vi "ParseObject.vi"(8 "error in (no error)":errorcluster, 10 "Tag In":string, 11 "Object_XML":string) -> (0 "error out":errorcluster, 3 "Array":T1[](array[typedef]))   [LabVIEW 2022 SP3, in "Object_Editor.lvlib" / "Object_Editor.lvclass"]
uses:
  Object_Editor.lvclass
  TreeItem.ctl
  ItemType.ctl
  <vilib>/xml/Load XML String.vi
  <vilib>/xml/Close Reference(Node).vi
  <vilib>/xml/NI_XML.lvlib
  <resource>/objmgr/DOMUserDefRef.rc
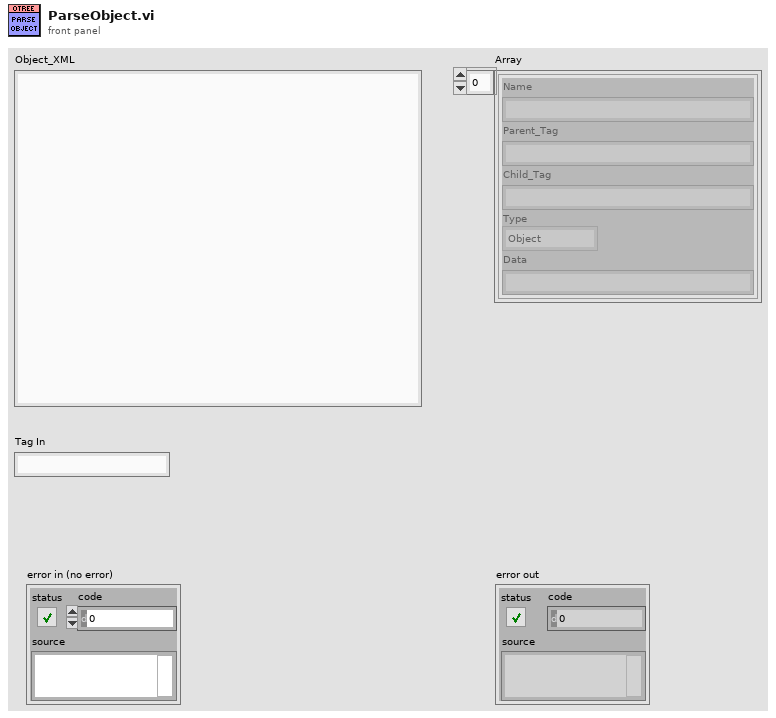
[diagram p1: front panel]
types:
  T1 = typedef "Object_Editor.lvlib/Object_Editor.lvclass/TreeItem.ctl" = cluster{"Name":string, "Parent_Tag":string, "Child_Tag":string, "Type":T2, "Data":string}
  T2 = typedef "Object_Editor.lvlib/Object_Editor.lvclass/ItemType.ctl" = enum16{"Object", "Ancestor"}
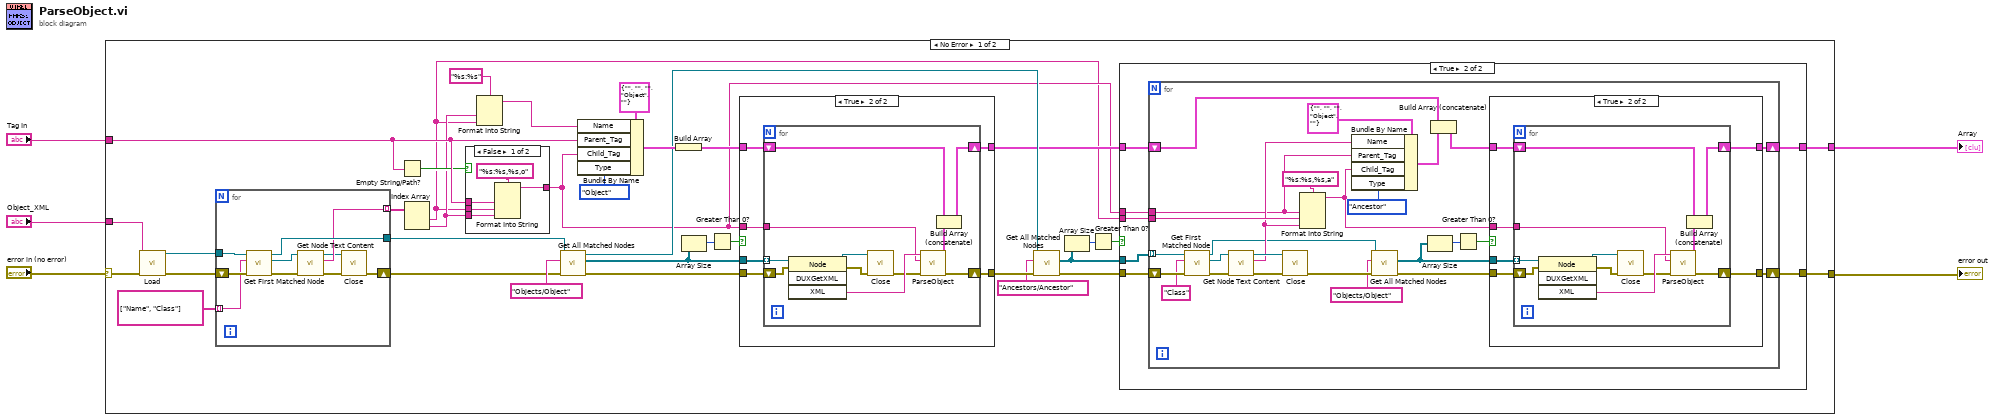
[diagram p0: block diagram]
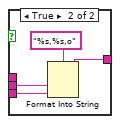
[diagram p4: hidden frame]
diagram:
  n1 = case shown="No Error" "error in (no error)" {
    selector: "error in (no error)" -> [w39 w132]
    tunnel: "Object_XML" -> [w38 _]
    tunnel: "Tag In" -> [w25 _]
    tunnel: [w12 w132] -> w1
    tunnel: [w11 _] -> w2
    frame No Error {
      n2 = call-poly <vilib>:"Load.vi"("XML string"=w38, "error in (no error)"=w39) -> ("DOM document out"=w36:refnum<k20>, "error out"=w37:errorcluster)  [unwired: 11 in, 1 out]
      n3 = for {
        tunnel: [w108] -> w30
        tunnel: [w107] -> w26 mode=indexing
        shift-right: [w104] -> w27
        shift-left: w37 -> [w112]
        tunnel: w36 -> [w111]
        tunnel: string[] ["Name", "Class"] -> [w106] mode=indexing
        n4 = call <vilib>:"Get First Matched Node.vi"("error in (no error)"=w112, "XPath expression"=w106, "node in"=w111) -> ("error out"=w110:errorcluster, "node result"=w109:refnum<k20>, "node out"=w108:refnum<k20>)  [unwired: 6 in]
        n5 = call <vilib>:"Get Node Text Content.vi"("error in (no error)"=w110, "node in"=w109) -> ("error out"=w105:errorcluster, "node text"=w107:string, "node out"=w103:refnum<k20>)  [unwired: 7 in]
        n6 = call-poly <vilib>:"Close.vi"("error in (no error)"=w105, "node"=w103) -> ("error out"=w104:errorcluster)  [unwired: 7 in]
      }
      n7 = Empty String/Path?(string/path=w25) -> (empty?=w24:bool)
      n8 = Index Array(array=w26) -> (element #1=w7:string, element #2=w8:string)  [unwired: 2 in]
      n9 = case shown="False" w24 {
        tunnel: [w97 w99] -> w14
        tunnel: w7 -> [w96 w101]
        tunnel: w8 -> [w95 w100]
        tunnel: w25 -> [w94 _]
        frame False {
          n10 = Format Into String(format string="%s:%s,%s,o", w94, w96, w95) -> (resulting string=w97:string)  [unwired: 2 in, 1 out]
        }
        frame True {
          n11 = Format Into String(format string="%s,%s,o", w101, w100) -> (resulting string=w99:string)  [unwired: 2 in, 1 out]
        }
      }
      n12 = Format Into String(format string="%s:%s", w8, w7) -> (resulting string=w6:string)  [unwired: 2 in, 1 out]
      n13 = call <vilib>:"Get All Matched Nodes.vi"("error in (no error)"=w27, "XPath expression"="Objects/Object", "node in"=w30) -> ("error out"=w34:errorcluster, "node result array"=w33:refnum<k20>[], "node out"=w20:refnum<k20>)  [unwired: 6 in]
      n14 = Bundle By Name(cluster=T1 {"Name"="", "Parent_Tag"="", "Child_Tag"="", "Type"=enum."Object", "Data"=""} ("Cluster"), "Name"=w6, "Parent_Tag"=w25, "Child_Tag"=w14, "Type"=ItemType."Object") -> (w23:T1)
      n15 = Build Array(w23) -> (w22:T1[])
      n16 = Array Size(array=w33) -> (size(s)=w32:i32)
      n17 = Greater Than 0?(x=w32) -> (x > 0?=w31:bool)
      n18 = case shown="True" w31 {
        tunnel: w34 -> [w113 w120]
        tunnel: w33 -> [_ w119]
        tunnel: w22 -> [w114 w115]
        tunnel: w14 -> [_ w118]
        tunnel: [w113 w117] -> w21
        tunnel: [w114 w116] -> w15
        frame False {
        }
        frame True {
          n19 = for {
            tunnel: w119 -> [w131] mode=indexing
            shift-right: [w129] -> w117
            shift-left: w120 -> [w130]
            shift-right: [w125] -> w116
            shift-left: w115 -> [w127]
            tunnel: w118 -> [w124]
            n20 = invoke class="Node" method="DUXGetXML"(reference=w131, error in=w130) -> (reference out=w121:refnum<k20>, error out=w123:errorcluster, "XML"=w128:string)  [unwired: 2 in, 1 out]
            n21 = call-poly <vilib>:"Close.vi"("error in (no error)"=w123, "node"=w121) -> ("error out"=w122:errorcluster)  [unwired: 7 in]
            n22 = call "ParseObject.vi"("error in (no error)"=w122, "Tag In"=w124, "Object_XML"=w128) -> ("error out"=w129:errorcluster, "Array"=w126:T1[])  [unwired: 7 in]
            n23 = Build Array (concatenate)(w127, w126) -> (w125:T1[])
          }
        }
      }
      n24 = call <vilib>:"Get All Matched Nodes.vi"("error in (no error)"=w21, "XPath expression"="Ancestors/Ancestor", "node in"=w20) -> ("error out"=w19:errorcluster, "node result array"=w17:refnum<k20>[])  [unwired: 6 in, 1 out]
      n25 = Array Size(array=w17) -> (size(s)=w18:i32)
      n26 = Greater Than 0?(x=w18) -> (x > 0?=w16:bool)
      n27 = case shown="True" w16 {
        tunnel: w19 -> [w41 w48]
        tunnel: w17 -> [_ w47]
        tunnel: [w41 w43] -> w12
        tunnel: w15 -> [w40 w44]
        tunnel: w14 -> [_ w46]
        tunnel: w7 -> [_ w45]
        tunnel: [w40 w42] -> w11
        frame False {
        }
        frame True {
          n28 = for {
            tunnel: w47 -> [w73] mode=indexing
            shift-right: [w50] -> w43
            shift-left: w48 -> [w74]
            tunnel: w46 -> [w64]
            tunnel: w45 -> [w66]
            shift-right: [w51] -> w42
            shift-left: w44 -> [w63]
            n29 = call <vilib>:"Get First Matched Node.vi"("error in (no error)"=w74, "XPath expression"="Class", "node in"=w73) -> ("error out"=w72:errorcluster, "node result"=w71:refnum<k20>, "node out"=w57:refnum<k20>)  [unwired: 6 in]
            n30 = call <vilib>:"Get Node Text Content.vi"("error in (no error)"=w72, "node in"=w71) -> ("error out"=w69:errorcluster, "node text"=w65:string, "node out"=w68:refnum<k20>)  [unwired: 7 in]
            n31 = call-poly <vilib>:"Close.vi"("error in (no error)"=w69, "node"=w68) -> ("error out"=w59:errorcluster)  [unwired: 7 in]
            n32 = Format Into String(format string="%s:%s,%s,a", w64, w66, w65) -> (resulting string=w53:string)  [unwired: 2 in, 1 out]
            n33 = Bundle By Name(cluster=T1 {"Name"="", "Parent_Tag"="", "Child_Tag"="", "Type"=enum."Object", "Data"=""} ("Cluster"), "Name"=w65, "Parent_Tag"=w64, "Child_Tag"=w53, "Type"=ItemType."Ancestor") -> (w62:T1)
            n34 = call <vilib>:"Get All Matched Nodes.vi"("error in (no error)"=w59, "XPath expression"="Objects/Object", "node in"=w57) -> ("error out"=w58:errorcluster, "node result array"=w55:refnum<k20>[])  [unwired: 6 in, 1 out]
            n35 = Array Size(array=w55) -> (size(s)=w60:i32)
            n36 = Build Array (concatenate)(w63, w62) -> (w54:T1[])
            n37 = Greater Than 0?(x=w60) -> (x > 0?=w56:bool)
            n38 = case shown="True" w56 {
              tunnel: w58 -> [w75 w82]
              tunnel: w55 -> [_ w81]
              tunnel: w54 -> [w76 w77]
              tunnel: w53 -> [_ w80]
              tunnel: [w75 w79] -> w50
              tunnel: [w76 w78] -> w51
              frame False {
              }
              frame True {
                n39 = for {
                  tunnel: w81 -> [w93] mode=indexing
                  shift-right: [w91] -> w79
                  shift-left: w82 -> [w92]
                  shift-right: [w87] -> w78
                  shift-left: w77 -> [w89]
                  tunnel: w80 -> [w86]
                  n40 = invoke class="Node" method="DUXGetXML"(reference=w93, error in=w92) -> (reference out=w83:refnum<k20>, error out=w85:errorcluster, "XML"=w90:string)  [unwired: 2 in, 1 out]
                  n41 = call-poly <vilib>:"Close.vi"("error in (no error)"=w85, "node"=w83) -> ("error out"=w84:errorcluster)  [unwired: 7 in]
                  n42 = call "ParseObject.vi"("error in (no error)"=w84, "Tag In"=w86, "Object_XML"=w90) -> ("error out"=w91:errorcluster, "Array"=w88:T1[])  [unwired: 7 in]
                  n43 = Build Array (concatenate)(w89, w88) -> (w87:T1[])
                }
              }
            }
          }
        }
      }
    }
    frame Error {
    }
  }
  "error out" <- w1
  "Array" <- w2
